vi "LVExampleServer.vi"() -> ()   [LabVIEW 2011]
uses:
  C:/Users/wasonj/Documents/CATS/RobotRaconteur/RobotRaconteur/LabView/lvexampleservice.dll
  lvexampleservice.dll
panel:
  in  "p1":dbl
  out "p2":dbl[](array[numeric])
  in  "stop":bool
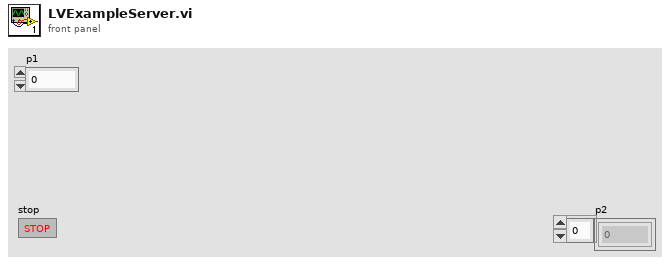
[diagram p1: front panel]
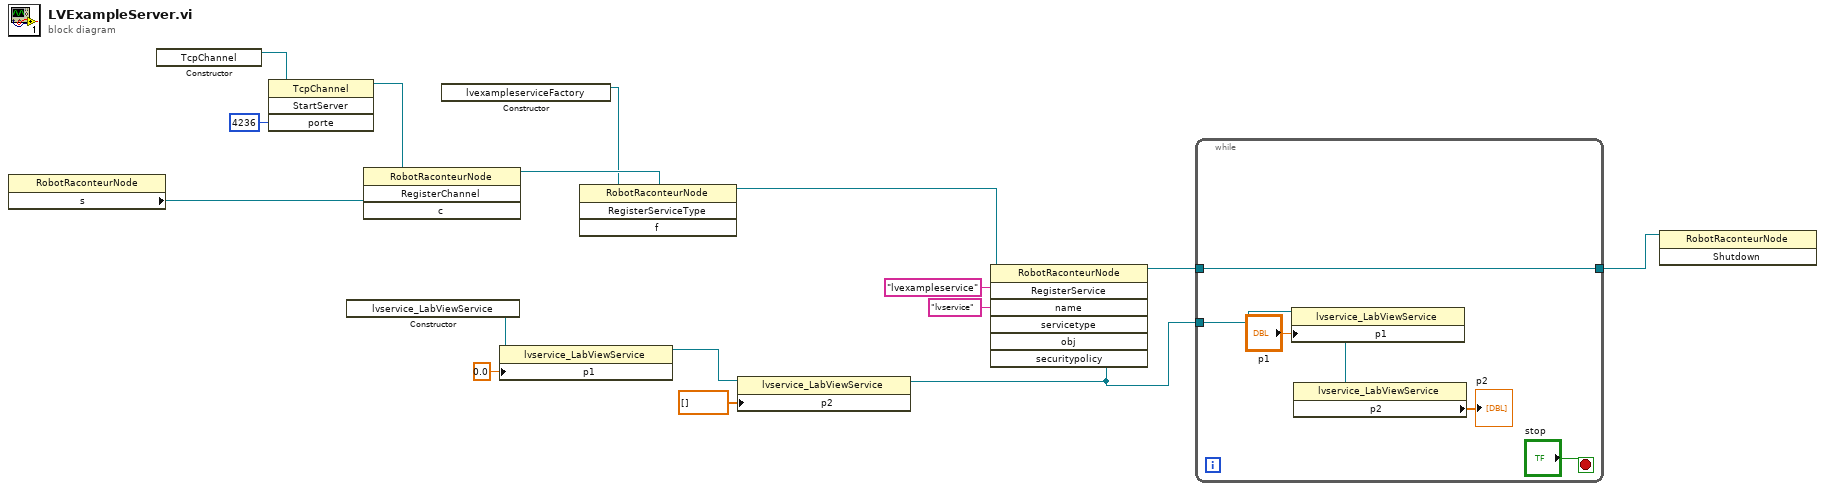
[diagram p0: block diagram]
diagram:
  n1 = property class="RobotRaconteurNode"() -> ("s"=w14:refnum<k24>)  [unwired: 2 in, 2 out]
  n2 = constructor class="TcpChannel"() -> (reference out=w16:refnum<k24>)  [unwired: 3 in, 2 out]
  n3 = invoke class="TcpChannel" method="StartServer"(reference=w16, "porte"=4236) -> (reference out=w13:refnum<k24>)  [unwired: 2 in, 3 out]
  n4 = constructor class="lvservice_LabViewService"() -> (reference out=w9:refnum<k24>)  [unwired: 3 in, 2 out]
  n5 = invoke class="RobotRaconteurNode" method="RegisterChannel"(reference=w14, "c"=w13) -> (reference out=w12:refnum<k24>)  [unwired: 2 in, 3 out]
  n6 = constructor class="lvexampleserviceFactory"() -> (reference out=w11:refnum<k24>)  [unwired: 3 in, 2 out]
  n7 = property class="lvservice_LabViewService"(reference=w9, "p1"=0.0) -> (reference out=w7:refnum<k24>)  [unwired: 1 in, 1 out]
  n8 = invoke class="RobotRaconteurNode" method="RegisterServiceType"(reference=w12, "f"=w11) -> (reference out=w10:refnum<k24>)  [unwired: 2 in, 3 out]
  n9 = property class="lvservice_LabViewService"(reference=w7, "p2"=dbl[] []) -> (reference out=w2:refnum<k24>)  [unwired: 1 in, 1 out]
  n10 = invoke class="RobotRaconteurNode" method="RegisterService"(reference=w10, "name"="lvservice", "servicetype"="lvexampleservice", "obj"=w2) -> (reference out=w4:refnum<k24>)  [unwired: 3 in, 6 out]
  n11 = while {
    tunnel: w4 -> [w21]
    tunnel: [w21] -> w3
    tunnel: w2 -> [w20]
    stop <- "stop" stop-if-true
    n12 = property class="lvservice_LabViewService"(reference=w20, "p1"="p1") -> (reference out=w18:refnum<k24>)  [unwired: 1 in, 1 out]
    n13 = property class="lvservice_LabViewService"(reference=w18) -> ("p2"=→"p2":dbl[])  [unwired: 1 in, 2 out]
  }
  n14 = invoke class="RobotRaconteurNode" method="Shutdown"(reference=w3) -> ()  [unwired: 2 in, 3 out]
